vi "P_IController.vi"() -> ()   [LabVIEW 2015]
panel:
  in  "Proportional":dbl=3.0
  in  "Integral":dbl
  in  "Coldfinger \nTemperature (K)":dbl=77.0
  in  "Temperature \nSetpoint":dbl=100.0
  in  "dt (s)":dbl=0.5 format="%#_13g"
  out "Temperature (K)":dbl
  out "?":dbl(graph)
  in  "?":bool
  out "Percentage \nHeater Output":dbl(slide) scale=0.0..100.0
  in  "Heater \nCurrent":u32(ring) items=["Low", "Medium", "High"]
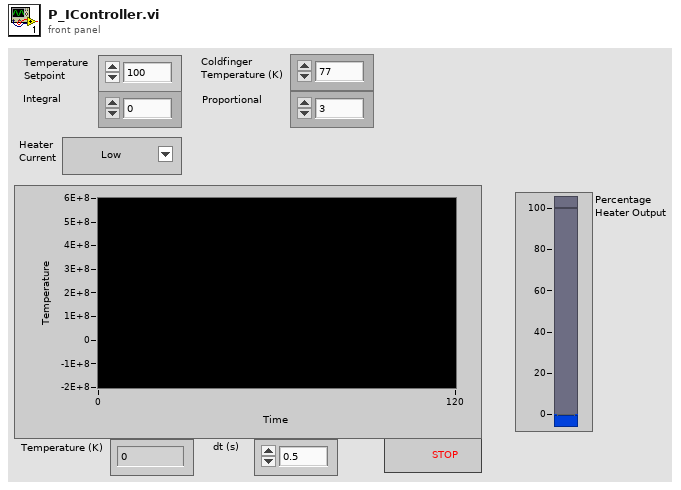
[diagram p1: front panel]
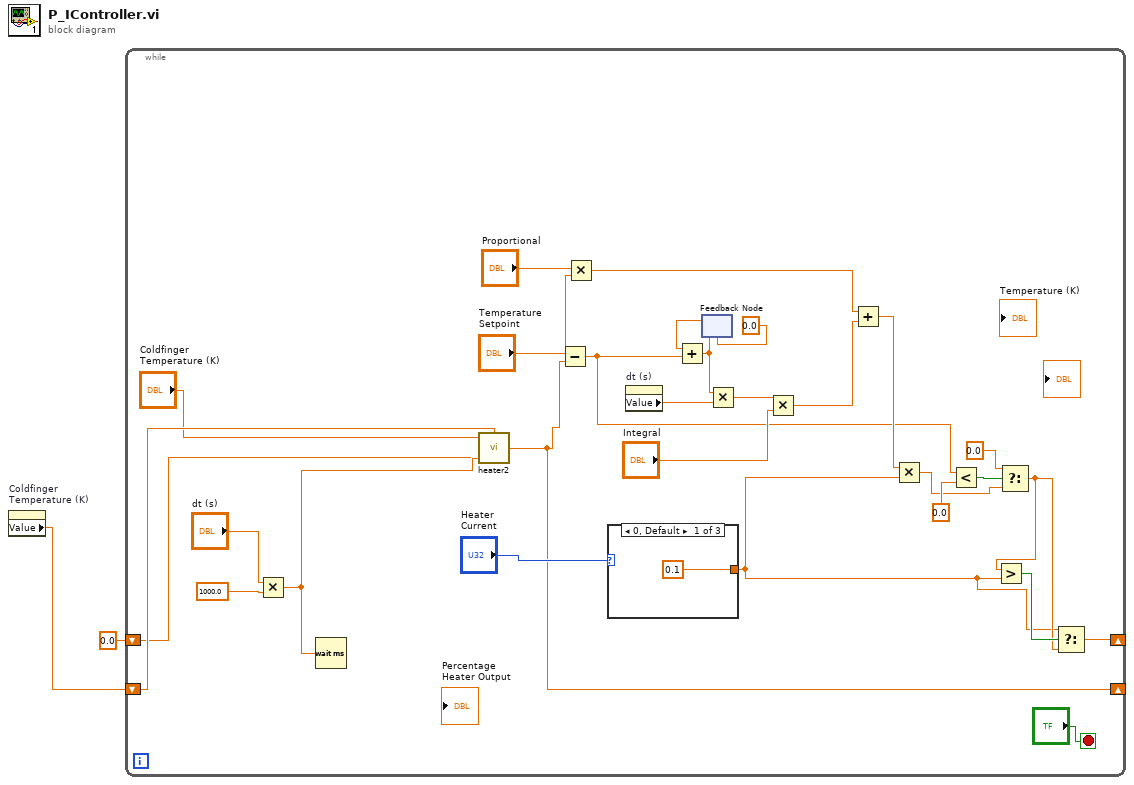
[diagram p0: block diagram]
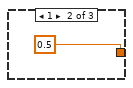
[diagram p2: hidden frame]
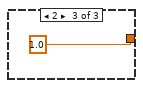
[diagram p3: hidden frame]
diagram:
  n1 = property on="Coldfinger \nTemperature (K)" class="DigNum (strict)"() -> ("Value"=w2:dbl)  [unwired: 2 in, 2 out]
  n2 = while {
    shift-right: [w4] -> _
    shift-left: w2 -> [w17]
    shift-right: [w7] -> _
    shift-left: 0.0 -> [w6]
    stop <- "?" stop-if-true
    n3 = Multiply(x="dt (s)", y=1000.0) -> (x*y=w8:dbl)
    n4 = Wait (ms)(milliseconds to wait=w8) -> ()  [unwired: 1 out]
    n5 = call "heater2.vi"("Tin"=w17, "dt (seconds)"=w8, "Current"=w6, "Tamb"="Coldfinger \nTemperature (K)") -> ("Tout"=w4:dbl)
    n6 = Subtract(x="Temperature \nSetpoint", y=w4) -> (x-y=w3:dbl)
    n7 = Multiply(x="Proportional", y=w3) -> (x*y=w19:dbl)
    n8 = case shown="0, Default" "Heater \nCurrent" {
      tunnel: [0.1 0.5 1.0] -> w5
      frame 0, Default {
      }
      frame 1 {
      }
      frame 2 {
      }
    }
    n9 = property on="dt (s)" class="DigNum (strict)"() -> ("Value"=w23:dbl)  [unwired: 2 in, 2 out]
    n10 = feedback #1(0.0 ("x+y")) -> (w25:dbl)
    n11 = Add(x=w25, y=w3) -> (x+y=w22:dbl)
    n12 = feedback-in #1(w22) -> ()
    n13 = Multiply(x=w22, y=w23) -> (x*y=w21:dbl)
    n14 = Multiply(x=w21, y="Integral") -> (x*y=w18:dbl)
    n15 = Add(x=w19, y=w18) -> (x+y=w16:dbl)
    n16 = Multiply(x=w16, y=w5) -> (x*y=w12:dbl)
    n17 = Less?(x=w3, y=0.0) -> (x < y?=w14:bool)
    n18 = Select(t=0.0, s=w14, f=w12) -> (s? t:f=w10:dbl)
    n19 = Greater?(x=w10, y=w5) -> (0:w11:bool)
    n20 = Select(t=w5, s=w11, f=w10) -> (s? t:f=w7:dbl)
  }
